vi "compass_aroplane.vi"(4 "center":cluster{"x":i32, "y":i32}, 6 "size":i16, 10 "pict in":picture) -> (3 "pict out":picture)   [LabVIEW 2017]
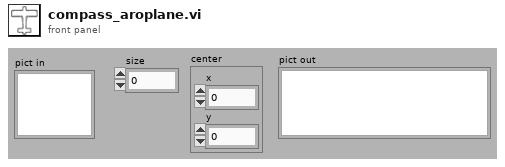
[diagram p1: front panel]
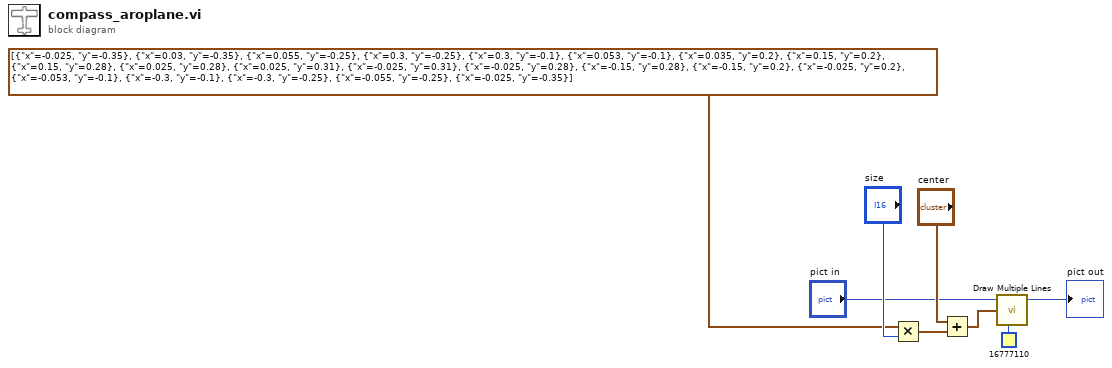
[diagram p0: block diagram]
diagram:
  n1 = Multiply(x=cluster{"x":dbl, "y":dbl}[] [{"x"=-0.025, "y"=-0.35}, {"x"=0.03, "y"=-0.35}, {"x"=0.055, "y"=-0.25}, {"x"=0.3, "y"=-0.25}, {"x"=0.3, "y"=-0.1}, {"x"=0.053, "y"=-0.1}, {"x"=0.035, "y"=0.2}, {"x"=0.15, "y"=0.2}, {"x"=0.15, "y"=0.28}, {"x"=0.025, "y"=0.28}, {"x"=0.025, "y"=0.31}, {"x"=-0.025, "y"=0.31}, {"x"=-0.025, "y"=0.28}, {"x"=-0.15, "y"=0.28}, {"x"=-0.15, "y"=0.2}, {"x"=-0.025, "y"=0.2}, {"x"=-0.053, "y"=-0.1}, {"x"=-0.3, "y"=-0.1}, {"x"=-0.3, "y"=-0.25}, {"x"=-0.055, "y"=-0.25}, {"x"=-0.025, "y"=-0.35}] ("line endpoints 2"), y="size") -> (x*y=w7:cluster{"x":dbl, "y":dbl}[])
  n2 = Add(x="center", y=w7) -> (x+y=w5:cluster{"x":dbl, "y":dbl}[])
  n3 = call <vilib>:"Draw Multiple Lines.vi"("picture"="pict in", "line endpoints"=w5, "color(black)"=u32 16777110) -> ("new picture"=→"pict out":picture)  [unwired: 6 in]
